vi "QueryTarget.vi"(8 "error in (no error)":errorcluster, 11 "Target Reference in":refnum<k39>) -> (0 "error out":errorcluster, 2 "Target Information":T1, 3 "Target Reference out":refnum<k39>)   [LabVIEW 2027, in "VeriStandTestUtilities.lvlib"]
uses:
  VeriStandTestUtilities.lvlib
  C:/NetCoreDLL/NationalInstruments.VeriStand.SystemDefinitionAPI.dll
  NetCoreDLL/NationalInstruments.VeriStand.SystemDefinitionAPI.dll
  TargetInformation.ctl
  ChassisInformation.ctl
panel:
  in  "Target Information":T1
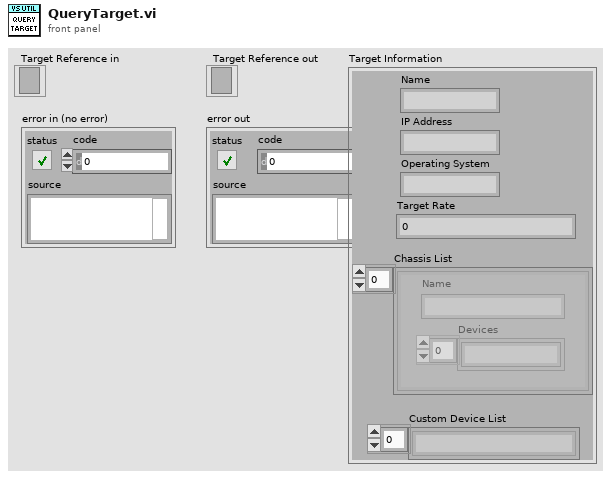
[diagram p1: front panel]
types:
  T1 = typedef "VeriStandTestUtilities.lvlib/TargetInformation.ctl" = cluster{"Name":string, "IP Address":string, "Operating System":string, "Target Rate":dbl, "Chassis List":T2[], "Custom Device List":string[]}
  T2 = typedef "VeriStandTestUtilities.lvlib/ChassisInformation.ctl" = cluster{"Name":string, "Devices":string[]}
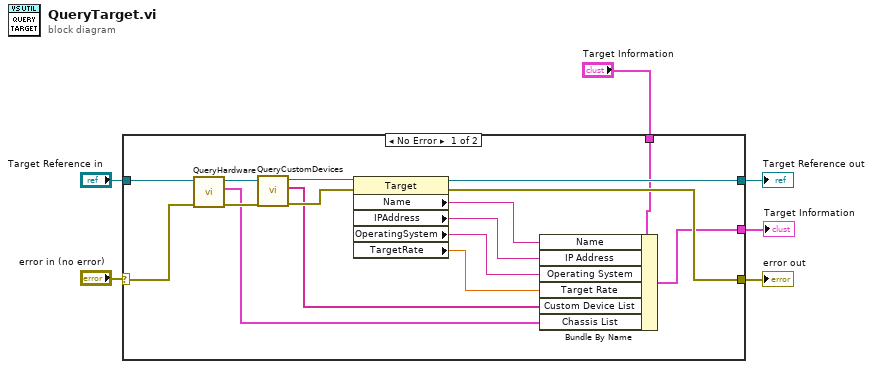
[diagram p0: block diagram]
diagram:
  n1 = case shown="No Error" "error in (no error)" {
    selector: "error in (no error)" -> [w21 w24]
    tunnel: [w22 w24] -> w5
    tunnel: "Target Reference in" -> [w13 w23]
    tunnel: [w20 w23] -> w3
    tunnel: "Target Information" -> [w19 _]
    tunnel: [w14 _] -> w1
    frame No Error {
      n2 = call "QueryHardware.vi"("error in (no error)"=w21, "NationalInstruments.VeriStand.SystemDefinitionAPI.Target"=w13) -> ("error out"=w10:errorcluster, "Chassis List out"=w7:T2[], "NationalInstruments.VeriStand.SystemDefinitionAPI.Target"=w12:refnum<k39>)  [unwired: 7 in]
      n3 = call "QueryCustomDevices.vi"("error in (no error)"=w10, "NationalInstruments.VeriStand.SystemDefinitionAPI.Target"=w12) -> ("error out"=w9:errorcluster, "Custom Devices"=w8:string[], "NationalInstruments.VeriStand.SystemDefinitionAPI.Target"=w11:refnum<k39>)  [unwired: 7 in]
      n4 = property class="Target"(reference=w11, error in=w9) -> (reference out=w20:refnum<k39>, error out=w22:errorcluster, "Name"=w18:string, "IPAddress"=w17:string, "OperatingSystem"=w16:string, "TargetRate"=w15:dbl)
      n5 = Bundle By Name(cluster=w19, "Name"=w18, "IP Address"=w17, "Operating System"=w16, "Target Rate"=w15, "Custom Device List"=w8, "Chassis List"=w7) -> (w14:T1)
    }
    frame Error {
    }
  }
  "error out" <- w5
  "Target Reference out" <- w3
  "Target Information" <- w1
